vi "set Active Object Transform.vi"(10 "Transform":T1, 11 "Scene in":refnum<class "Scene.lvclass">) -> (3 "Scene out":refnum<class "Scene.lvclass">)   [LabVIEW 2020, in "Application.lvlib" / "Scene.lvclass"]
uses:
  Scene.lvclass
  Libraries/3D/Vector 3D.ctl
  Libraries/3D/3D.lvlib
  Libraries/3D/Transform.ctl
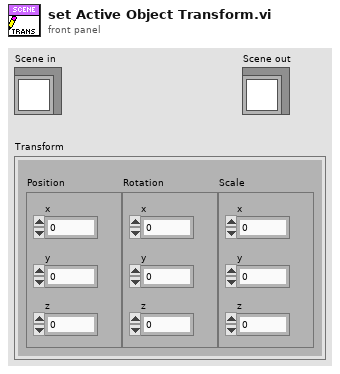
[diagram p1: front panel]
types:
  T1 = typedef "3D.lvlib/Transform.ctl" = cluster{"Position":T2, "Rotation":T2, "Scale":T2}
  T2 = typedef "3D.lvlib/Vector 3D.ctl" = cluster{"x":sgl, "y":sgl, "z":sgl}
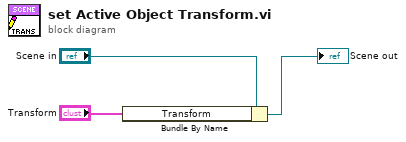
[diagram p0: block diagram]
diagram:
  n1 = Bundle By Name(cluster="Scene in", "Transform"="Transform") -> (→"Scene out":refnum<class "Scene.lvclass">)
